vi "Boiler Controller.vi"(8 "error in (no error)":errorcluster, 11 "Message Queues":T1) -> (0 "error out":errorcluster)   [LabVIEW 2015]
uses:
  support/Message Queue/All Message Queues.ctl
  support/Message Queue/Message Cluster.ctl
  support/Message Queue/Message Queue.lvlib
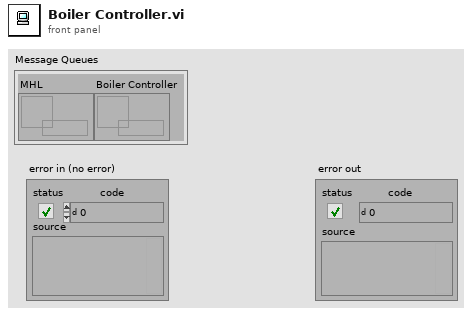
[diagram p1: front panel]
types:
  T1 = typedef "Message Queue.lvlib/All Message Queues.ctl" = cluster{"MHL":refnum<queue>, "Boiler Controller":refnum<queue>}
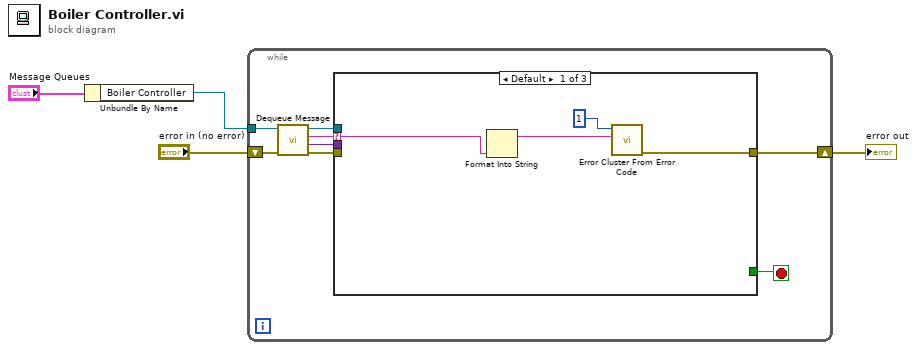
[diagram p0: block diagram]
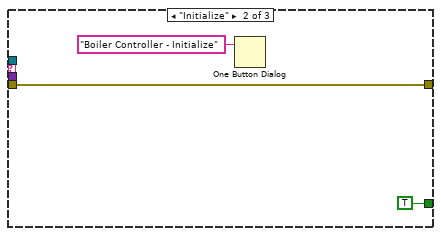
[diagram p2: hidden frame]
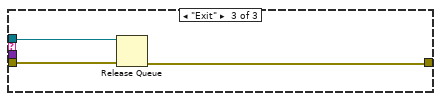
[diagram p3: hidden frame]
diagram:
  n1 = Unbundle By Name("Message Queues") -> ("Boiler Controller"=w3:refnum<queue>)
  n2 = while {
    tunnel: w3 -> [w12]
    shift-right: [w6] -> w1
    shift-left: "error in (no error)" -> [w9]
    stop <- w5 stop-if-true
    n3 = call "Dequeue Message.vi"("error in (no error)"=w9, "Message Queue"=w12) -> ("error out"=w10:errorcluster, "Message Data"=w11:variant, "Message"=w8:string, "dup Message Queue"=w7:refnum<queue>)  [unwired: 6 in]
    n4 = case shown="Default" w8 {
      selector: w8 -> [w13 _ _]
      tunnel: w10 -> [_ w18 w21]
      tunnel: w11 -> [_ _ _]
      tunnel: w7 -> [_ _ w22]
      tunnel: [w16 w18 w20] -> w6
      tunnel: [_ TRUE _] -> w5
      frame Default {
        n5 = Format Into String(w13) -> (resulting string=w14:string)  [unwired: 3 in, 1 out]
        n6 = call <vilib>:"Error Cluster From Error Code.vi"("error message (\"\")"=w14, "error code (0)"=1) -> ("error out"=w16:errorcluster)  [unwired: 7 in]
      }
      frame "Initialize" {
        n7 = One Button Dialog(message="Boiler Controller - Initialize") -> ()  [unwired: 1 in, 1 out]
      }
      frame "Exit" {
        n8 = Release Queue(queue=w22, error in (no error)=w21) -> (error out=w20:errorcluster)  [unwired: 1 in, 2 out]
      }
    }
  }
  "error out" <- w1
